vi "Test.vi"   [LabVIEW 2017]
doc: "This VI starts when test mode begins, and will automatically be terminated when it ends. It will automatically publish I/O values, and you can add manual tests that can be invoked from the dashboard."
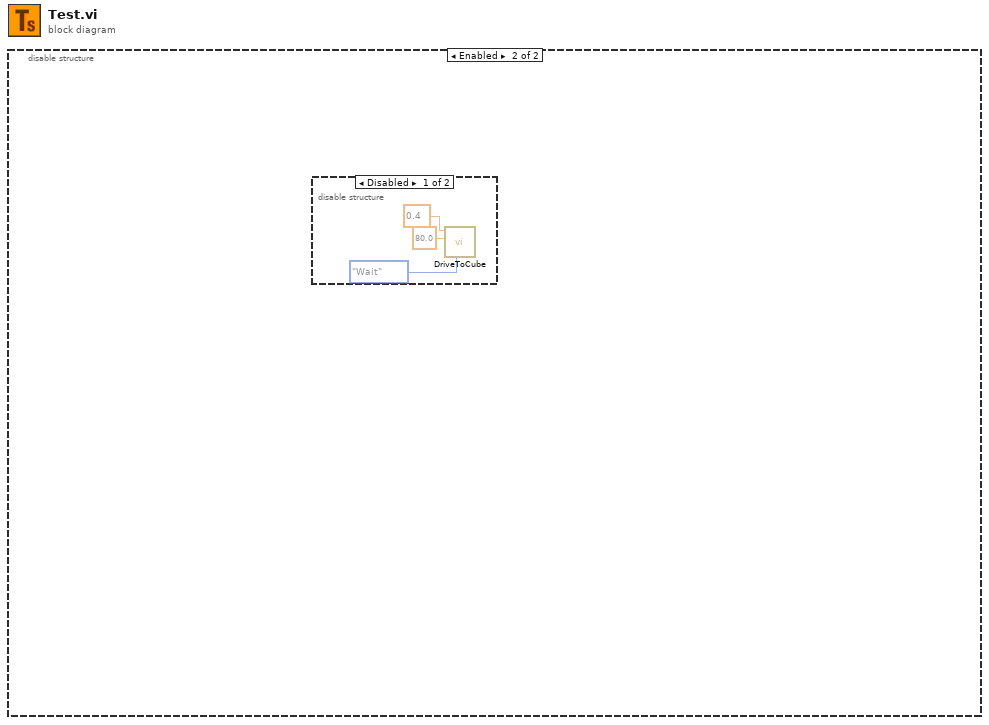
[diagram p0: block diagram]
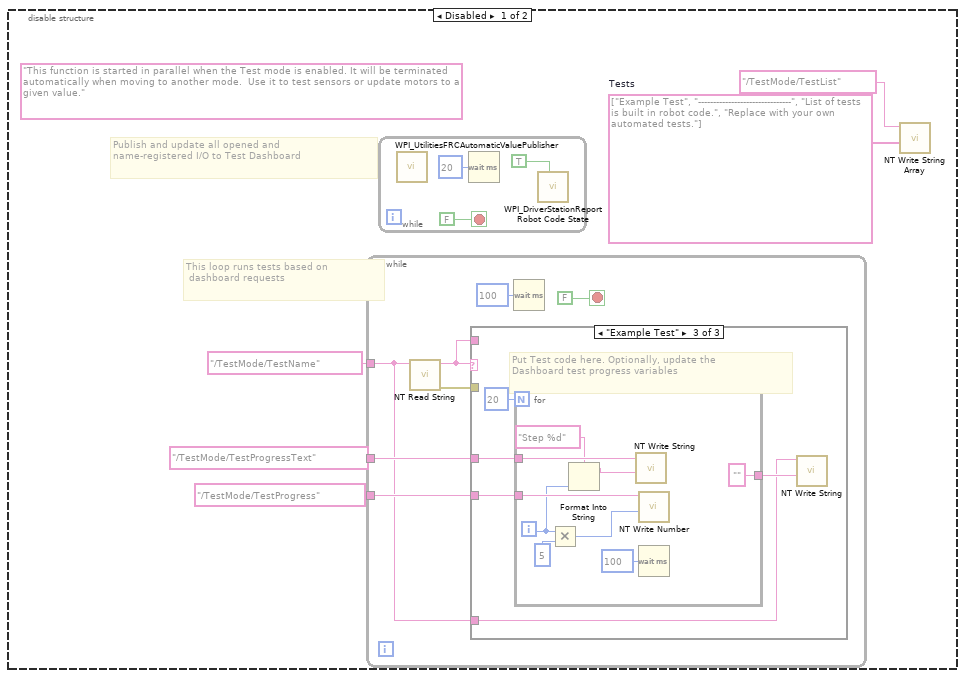
[diagram p2: hidden frame]
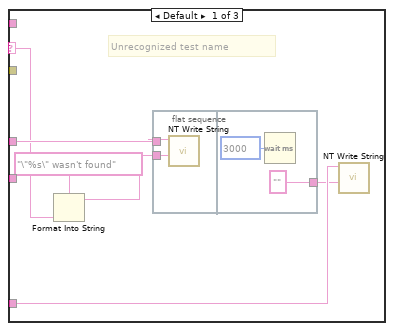
[diagram p3: hidden frame]
diagram:
  n1 = disable-structure shown="Enabled" {
    frame Disabled {
      w2 = string[] ["Example Test", "-------------------------------", "List of tests is built in robot code.", "Replace with your own automated tests."]  # Tests
      (unwired) "This function is started in parallel when the Test mode is enabled. It will be terminated automatically when moving to another mode.  Use it to test sensors or update motors to a given value."
      # "This loop runs tests based on \n dashboard requests"
      # "Publish and update all opened and\nname-registered I/O to Test Dashboard"
      n2 = while {
        tunnel: "/TestMode/TestName" ("Name") -> [w10]
        tunnel: "/TestMode/TestProgressText" ("Name") -> [w13]
        tunnel: "/TestMode/TestProgress" ("Name") -> [w12]
        stop <- FALSE stop-if-true
        n3 = call <vilib>:"NT Read String.vi"("Name"=w10) -> ("error out"=w9:errorcluster, "String"=w11:string)  [unwired: 9 in]
        n4 = case shown="\"Example Test\"" w11 {
          selector: w11 -> [w20 _ _]
          tunnel: w10 -> [w17 _ w26]
          tunnel: w13 -> [w21 _ w29]
          tunnel: w12 -> [_ _ w30]
          tunnel: w11 -> [_ _ _]
          tunnel: w9 -> [_ _ _]
          frame Default {
            # "Unrecognized test name"
            n5 = Format Into String(format string="\"%s\" wasn't found" ("Name"), w20) -> (resulting string=w19:string)  [unwired: 2 in, 1 out]
            n6 = flat-sequence {
              tunnel: w21 -> [w22]
              tunnel: w19 -> [w23]
              tunnel: ["" ("Name")] -> w16
              frame #0 {
                n7 = call <vilib>:"NT Write String.vi"("String"=w23, "Name"=w22) -> ()  [unwired: 9 in, 1 out]
              }
              frame #1 {
                n8 = Wait (ms)(milliseconds to wait=u32 3000) -> ()  [unwired: 1 out]
              }
            }
            n9 = call <vilib>:"NT Write String.vi"("String"=w16, "Name"=w17) -> ()  [unwired: 9 in, 1 out]
          }
          frame "" {
            # "No test to run"
          }
          frame "Example Test" {
            # "Put Test code here. Optionally, update the\nDashboard test progress variables"
            n10 = for {
              N: 20 -> [_]
              tunnel: w30 -> [w39]
              tunnel: w29 -> [w37]
              tunnel: ["" ("String")] -> w27
              i -> [w34]
              n11 = Multiply(x=w34, y=u32 5 ("milliseconds to wait")) -> (x*y=w35:u32)
              n12 = Format Into String(format string="Step %d", w34) -> (resulting string=w32:string)  [unwired: 2 in, 1 out]
              n13 = call <vilib>:"NT Write String.vi"("String"=w32, "Name"=w37) -> ()  [unwired: 9 in, 1 out]
              n14 = call <vilib>:"NT Write Number.vi"("Numeric"=w35, "Name"=w39) -> ()  [unwired: 9 in, 1 out]
              n15 = Wait (ms)(milliseconds to wait=u32 100) -> ()  [unwired: 1 out]
            }
            n16 = call <vilib>:"NT Write String.vi"("String"=w27, "Name"=w26) -> ()  [unwired: 9 in, 1 out]
          }
        }
        n17 = Wait (ms)(milliseconds to wait=u32 100) -> ()  [unwired: 1 out]
      }
      n18 = while {
        stop <- FALSE stop-if-true
        n19 = call <vilib>:"WPI_UtilitiesFRCAutomaticValuePublisher.vi"() -> ()  [unwired: 12 in]
        n20 = Wait (ms)(milliseconds to wait=u32 20) -> ()  [unwired: 1 out]
        n21 = call <vilib>:"WPI_DriverStationReport Robot Code State.vi"("Test"=TRUE ("Autonomous")) -> ()  [unwired: 10 in, 1 out]
      }
      n22 = call <vilib>:"NT Write String Array.vi"("String Array"=w2, "Name"="/TestMode/TestList") -> ()  [unwired: 9 in, 1 out]
    }
    frame Enabled {
      n23 = disable-structure shown="Disabled" {
        frame Disabled {
          n24 = call "DriveToCube.vi"("Synchronication"=enum16{"Start", "Wait"}."Wait", "Distance"=80.0, "Speed"=0.4) -> ()  [unwired: 8 in, 1 out]
        }
        frame Enabled {
        }
      }
    }
  }
